vi "_Switch Lens Property Unit.vi"(5 "Lens Property In":T2={"Unit"=TRUE, "Count1"=1.0, "Count2"=1.0, "Step Size"=1.0}, 7 "Configuration":T1) -> (0 "DAC Value":i32=1, 1 "Step Size":dbl=1.0, 2 "Count2":dbl=1.0 caption="Stop", 3 "Count1":dbl=1.0 caption="Start")   [LabVIEW 2012]
uses:
  Type/_RT Configuration 2.ctl
  _Global Configuration.vi
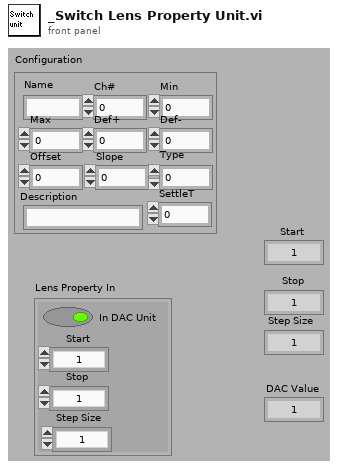
[diagram p1: front panel]
types:
  T1 = typedef "_RT Configuration 2.ctl" = cluster{"Name":string, "Ch#":u8, "Min":dbl, "Max":dbl, "Def+":dbl, "Def-":dbl, "Offset":dbl, "Slope":dbl, "Type":u8, "Description":string, "SettleT":dbl}
  T2 = cluster{"Unit":bool, "Count1":dbl, "Count2":dbl, "Step Size":dbl}
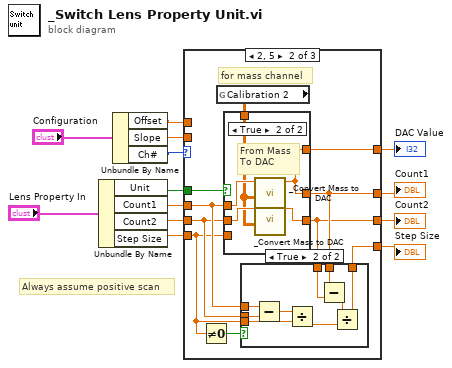
[diagram p0: block diagram]
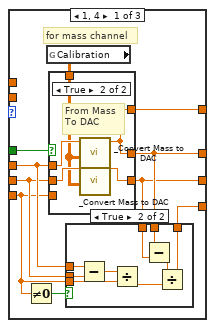
[diagram p2: hidden frame]
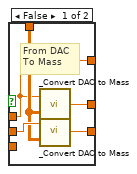
[diagram p4: hidden frame]
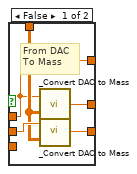
[diagram p6: hidden frame]
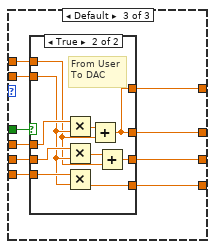
[diagram p7: hidden frame]
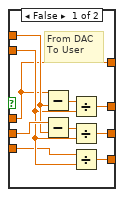
[diagram p8: hidden frame]
diagram:
  # "Always assume positive scan"
  n1 = Unbundle By Name("Lens Property In") -> ("Unit"=w7:bool, "Count1"=w13:dbl, "Count2"=w12:dbl, "Step Size"=w11:dbl)
  n2 = Unbundle By Name("Configuration") -> ("Offset"=w10:dbl, "Slope"=w9:dbl, "Ch#"=w3:u8)
  n3 = case shown="2, 5" w3 {
    tunnel: w13 -> [w20 w50 w83]
    tunnel: w12 -> [w19 w49 w82]
    tunnel: w11 -> [w18 w48 w81]
    tunnel: w10 -> [_ _ w80]
    tunnel: w9 -> [_ _ w79]
    tunnel: w7 -> [w23 w53 w78]
    tunnel: [w17 w47 w77] -> w6
    tunnel: [w16 w46 w76] -> w5
    tunnel: [w22 w52 w75] -> w4
    tunnel: [w14 w44 w74] -> w2
    frame 1, 4 {
      # "for mass channel"
      n4 = Not Equal To 0?(x=w18) -> (x != 0?=w21:bool)
      n5 = global read "_Global Configuration.vi" "Calibration"() -> (w15:dbl[][])
      n6 = case shown="True" w23 {
        tunnel: w20 -> [w34 w43]
        tunnel: w19 -> [w38 w42]
        tunnel: [w37 w39] -> w17
        tunnel: [w36 w41] -> w16
        tunnel: w18 -> [_ _]
        tunnel: w15 -> [w35 w40]
        tunnel: [w34 w39] -> w14
        frame False {
          # "From DAC\nTo Mass"
          n7 = call "_Convert DAC to Mass.vi"("Calibration Table"=w35, "DAC"=w34) -> ("Mass"=w37:dbl)
          n8 = call "_Convert DAC to Mass.vi"("Calibration Table"=w35, "DAC"=w38) -> ("Mass"=w36:dbl)
        }
        frame True {
          # "From Mass\nTo DAC"
          n9 = call "_Convert Mass to DAC.vi"("Calibration Table"=w40, "Mass"=w43) -> ("DAC Value"=w39:dbl)  [unwired: 2 in, 3 out]
          n10 = call "_Convert Mass to DAC.vi"("Calibration Table"=w40, "Mass"=w42) -> ("DAC Value"=w41:dbl)  [unwired: 2 in, 3 out]
        }
      }
      n11 = case shown="True" w21 {
        tunnel: [w24 w30] -> w22
        tunnel: w20 -> [_ w29]
        tunnel: w19 -> [_ w28]
        tunnel: w18 -> [w24 w27]
        tunnel: w17 -> [_ w26]
        tunnel: w16 -> [_ w25]
        frame False {
        }
        frame True {
          n12 = Subtract(x=w29, y=w28) -> (x-y=w31:dbl)
          n13 = Divide(x=w31, y=w27) -> (x/y=w33:dbl)
          n14 = Subtract(x=w26, y=w25) -> (x-y=w32:dbl)
          n15 = Divide(x=w32, y=w33) -> (x/y=w30:dbl)
        }
      }
    }
    frame 2, 5 {
      # "for mass channel"
      n16 = Not Equal To 0?(x=w48) -> (x != 0?=w51:bool)
      n17 = global read "_Global Configuration.vi" "Calibration 2"() -> (w45:dbl[][])
      n18 = case shown="True" w53 {
        tunnel: w50 -> [w64 w73]
        tunnel: w49 -> [w68 w72]
        tunnel: [w67 w69] -> w47
        tunnel: [w66 w71] -> w46
        tunnel: w48 -> [_ _]
        tunnel: w45 -> [w65 w70]
        tunnel: [w64 w69] -> w44
        frame False {
          # "From DAC\nTo Mass"
          n19 = call "_Convert DAC to Mass.vi"("Calibration Table"=w65, "DAC"=w64) -> ("Mass"=w67:dbl)
          n20 = call "_Convert DAC to Mass.vi"("Calibration Table"=w65, "DAC"=w68) -> ("Mass"=w66:dbl)
        }
        frame True {
          # "From Mass\nTo DAC"
          n21 = call "_Convert Mass to DAC.vi"("Calibration Table"=w70, "Mass"=w73) -> ("DAC Value"=w69:dbl)  [unwired: 2 in, 3 out]
          n22 = call "_Convert Mass to DAC.vi"("Calibration Table"=w70, "Mass"=w72) -> ("DAC Value"=w71:dbl)  [unwired: 2 in, 3 out]
        }
      }
      n23 = case shown="True" w51 {
        tunnel: [w54 w60] -> w52
        tunnel: w50 -> [_ w59]
        tunnel: w49 -> [_ w58]
        tunnel: w48 -> [w54 w57]
        tunnel: w47 -> [_ w56]
        tunnel: w46 -> [_ w55]
        frame False {
        }
        frame True {
          n24 = Subtract(x=w59, y=w58) -> (x-y=w61:dbl)
          n25 = Divide(x=w61, y=w57) -> (x/y=w63:dbl)
          n26 = Subtract(x=w56, y=w55) -> (x-y=w62:dbl)
          n27 = Divide(x=w62, y=w63) -> (x/y=w60:dbl)
        }
      }
    }
    frame Default {
      n28 = case shown="True" w78 {
        tunnel: w83 -> [w84 w98]
        tunnel: w82 -> [w90 w99]
        tunnel: [w92 w94] -> w77
        tunnel: [w89 w100] -> w76
        tunnel: w80 -> [w87 w96]
        tunnel: w79 -> [w86 w97]
        tunnel: [w88 w95] -> w75
        tunnel: w81 -> [w85 w101]
        tunnel: [w84 w94] -> w74
        frame False {
          # "From DAC\nTo User"
          n29 = Subtract(x=w84, y=w87) -> (x-y=w93:dbl)
          n30 = Subtract(x=w90, y=w87) -> (x-y=w91:dbl)
          n31 = Divide(x=w93, y=w86) -> (x/y=w92:dbl)
          n32 = Divide(x=w91, y=w86) -> (x/y=w89:dbl)
          n33 = Divide(x=w85, y=w86) -> (x/y=w88:dbl)
        }
        frame True {
          # "From User\nTo DAC"
          n34 = Multiply(x=w98, y=w97) -> (x*y=w102:dbl)
          n35 = Multiply(x=w99, y=w97) -> (x*y=w103:dbl)
          n36 = Multiply(x=w101, y=w97) -> (x*y=w95:dbl)
          n37 = Add(x=w102, y=w96) -> (x+y=w94:dbl)
          n38 = Add(x=w103, y=w96) -> (x+y=w100:dbl)
        }
      }
    }
  }
  "Count1" <- w6
  "Count2" <- w5
  "Step Size" <- w4
  "DAC Value" <- w2
